vi "ReadParam.vi"(8 "error in (no error)":errorcluster caption="错误输入（无错误）", 10 "机种":string, 11 "路径":path) -> (0 "error out":errorcluster, 1 "Points":dbl[][](array[numeric]), 2 "Steps":dbl[][](array[numeric]), 3 "TemPath":path)   [LabVIEW 2016]
uses:
  <vilib>/Utility/config.llb/Read Key (String).vi
  <vilib>/Utility/config.llb/NI_LVConfig.lvlib
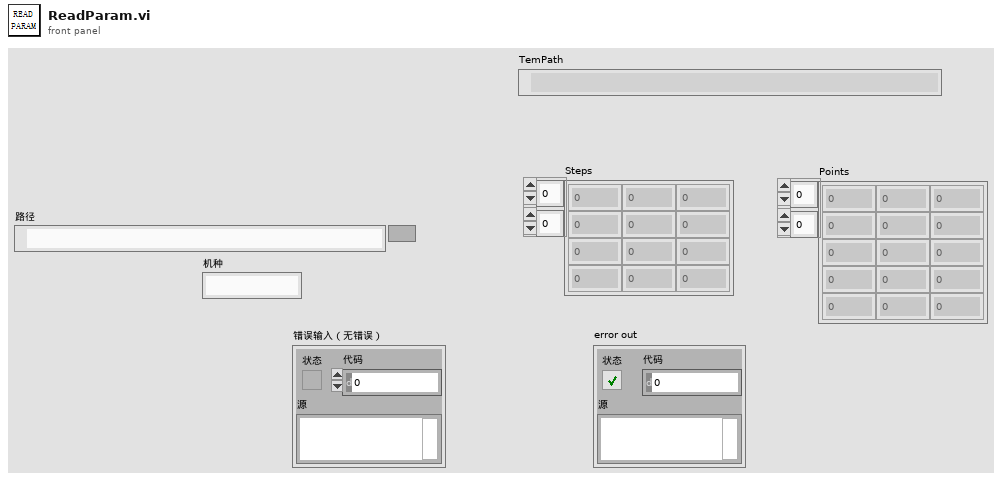
[diagram p1: front panel]
types:
  T1 = typedef "NI_LVConfig.lvlib/Config Data RefNum.ctl" = refnum<k1>
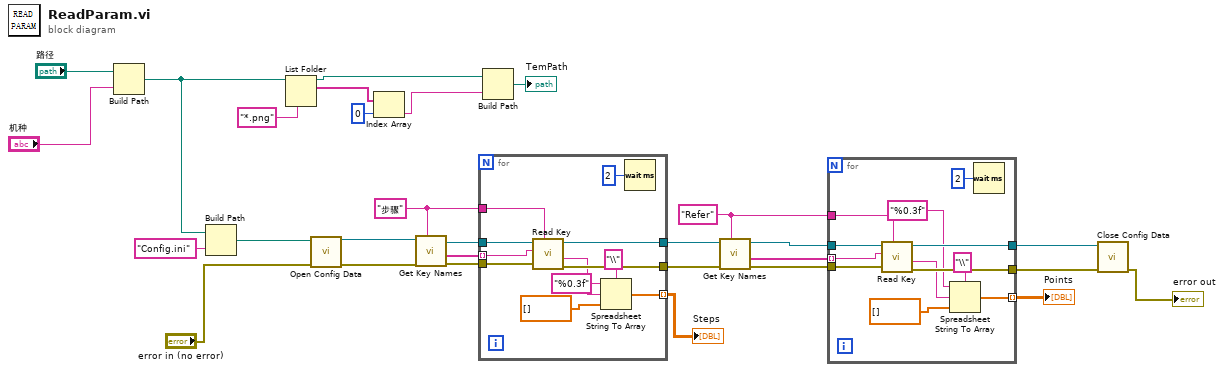
[diagram p0: block diagram]
diagram:
  w13 = "Refer" ("section")
  w20 = "步骤" ("section")
  n1 = Build Path(base path="路径", name or relative path="机种") -> (appended path=w4:path)
  n2 = Build Path(base path=w4, name or relative path="Config.ini" ("名称或相对路径")) -> (appended path=w26:path)
  n3 = List Folder(path=w4, pattern="*.png" ("类型")) -> (path out=w3:path, filenames=w6:string[])  [unwired: 2 in, 2 out]
  n4 = call <vilib>:"Open Config Data.vi"("error in (no error)"="error in (no error)", "configuration file path"=w26) -> ("error out"=w24:errorcluster, "refnum"=w25:T1)  [unwired: 7 in, 1 out]
  n5 = Index Array(array=w6, index=0 ("索引")) -> (element=w2:string)
  n6 = call <vilib>:"Get Key Names.vi"("section"=w20, "error in (no error)"=w24, "refnum"=w25) -> ("error out"=w21:errorcluster, "key names"=w19:string[], "refnum out"=w22:T1)  [unwired: 5 in, 1 out]
  n7 = for {
    tunnel: w22 -> [w41]
    tunnel: w21 -> [w40]
    tunnel: w20 -> [w39]
    tunnel: w19 -> [w38] mode=indexing
    tunnel: [w36] -> w18
    tunnel: [w35] -> w17
    tunnel: [w31] -> w12 mode=indexing
    n8 = call-poly <vilib>:"Read Key.vi"("section"=w39, "error in (no error)"=w40, "key"=w38, "refnum"=w41) -> ("error out"=w36:errorcluster, "value"=w34:string, "refnum out"=w35:T1)  [unwired: 4 in, 1 out]
    n9 = Spreadsheet String To Array(delimiter (Tab)="\\" ("分隔符(Tab)"), format string="%0.3f" ("格式字符串"), spreadsheet string=w34, array type (2D Dbl)=dbl[] [] ("数组类型(2D Dbl)")) -> (array=w31:dbl[])
    n10 = Wait (ms)(milliseconds to wait=u32 2 ("等待时间（毫秒）")) -> ()  [unwired: 1 out]
  }
  "Steps" <- w12
  n11 = Build Path(base path=w3, name or relative path=w2) -> (appended path=→"TemPath":path)
  n12 = call <vilib>:"Get Key Names.vi"("section"=w13, "error in (no error)"=w18, "refnum"=w17) -> ("error out"=w15:errorcluster, "key names"=w14:string[], "refnum out"=w16:T1)  [unwired: 5 in, 1 out]
  n13 = for {
    tunnel: w16 -> [w53]
    tunnel: w15 -> [w52]
    tunnel: w13 -> [w51]
    tunnel: w14 -> [w50] mode=indexing
    tunnel: [w48] -> w10
    tunnel: [w47] -> w9
    tunnel: [w43] -> w11 mode=indexing
    n14 = call-poly <vilib>:"Read Key.vi"("section"=w51, "error in (no error)"=w52, "key"=w50, "refnum"=w53) -> ("error out"=w48:errorcluster, "value"=w46:string, "refnum out"=w47:T1)  [unwired: 4 in, 1 out]
    n15 = Spreadsheet String To Array(delimiter (Tab)="\\" ("分隔符(Tab)"), format string="%0.3f" ("格式字符串"), spreadsheet string=w46, array type (2D Dbl)=dbl[] [] ("数组类型(2D Dbl)")) -> (array=w43:dbl[])
    n16 = Wait (ms)(milliseconds to wait=u32 2 ("等待时间（毫秒）")) -> ()  [unwired: 1 out]
  }
  "Points" <- w11
  n17 = call <vilib>:"Close Config Data.vi"("error in (no error)"=w10, "refnum"=w9) -> ("error out"=→"error out":errorcluster)  [unwired: 8 in, 1 out]
